vi "SubVI_Read_Allan_Result_TDMS.vi"() -> ()   [LabVIEW 2024]
panel:
  out "error out":errorcluster caption="错误输出"
  out "TDMS回放Allan偏差曲线":cluster{"Y":dbl[], "Y":dbl[]}(graph)
  in  "文件路径":path=path "D:/EG_FPGA_Project/Project/Labview_Output/allan_main_result.tdms"
  in  "error in":errorcluster caption="错误输入"
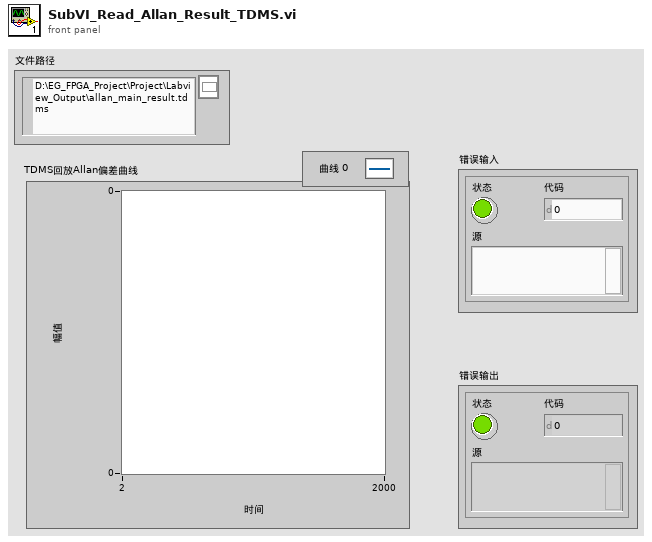
[diagram p1: front panel]
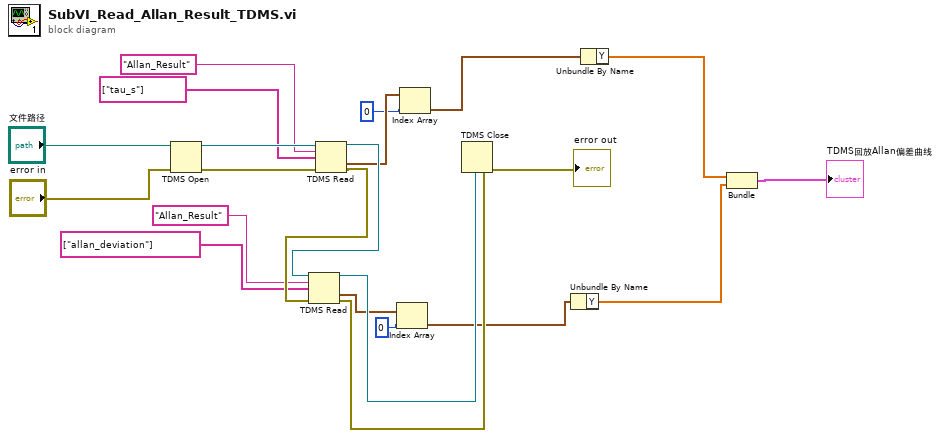
[diagram p0: block diagram]
diagram:
  n1 = TDMS Open(8:"error in", 11:"文件路径") -> (0:w18:errorcluster, 3:w22:refnum<k34>)  [unwired: 5 in]
  n2 = TDMS Read(0:w22, 5:"Allan_Result" ("组名称输入"), 7:string[] ["tau_s"] ("通道名称输入"), 11:w18) -> (4:w20:refnum<k34>, 10:w10:waveform(dbl)[], 15:w17:errorcluster)  [unwired: 4 in, 3 out]
  n3 = TDMS Read(0:w20, 5:"Allan_Result" ("组名称输入"), 7:string[] ["allan_deviation"] ("通道名称输入"), 11:w17) -> (4:w21:refnum<k34>, 10:w7:waveform(dbl)[], 15:w16:errorcluster)  [unwired: 4 in, 3 out]
  n4 = Index Array(array=w7, index=0 ("索引")) -> (element=w5:waveform(dbl))
  n5 = Index Array(array=w10, index=0 ("索引")) -> (element=w8:waveform(dbl))
  n6 = TDMS Close(8:w16, 11:w21) -> (0:→"error out":errorcluster)  [unwired: 1 out]
  n7 = Unbundle By Name(w5) -> ("Y"=w3:dbl[])
  n8 = Unbundle By Name(w8) -> ("Y"=w4:dbl[])
  n9 = Bundle("Y"=w4, "Y"=w3) -> (→"TDMS回放Allan偏差曲线":cluster{"Y":dbl[], "Y":dbl[]})  [unwired: 1 in]
